vi "Request Data.vi"(6 "Qualifier":string, 8 "error in":errorcluster, 9 "notifier":refnum<notifier>, 10 "Data to Send":string, 11 "Electronic Load in":refnum<class "Electronic Load.lvclass">) -> (0 "error out":errorcluster, 3 "Electronic Load out":refnum<class "Electronic Load.lvclass">)   [LabVIEW 2019, in "Electronic Load.lvlib" / "Electronic Load.lvclass"]
uses:
  Library/Electronic Load.lvclass
  C:/Users/Public/Documents/Development/builds/Instruments/Instruments.lvlibp/Library/Instruments.lvclass
  Library/Electronic Load.lvclass/Electronic Load.ctl
  Accessors/Read Available Channels.vi
  builds/Instruments/Instruments.lvlibp/Accessors/Read Measured.vi
  builds/Instruments/Instruments.lvlibp/Accessors/Read Snapshot.vi
  builds/Instruments/Instruments.lvlibp/Private/Accessors/Read Poll(ms).vi
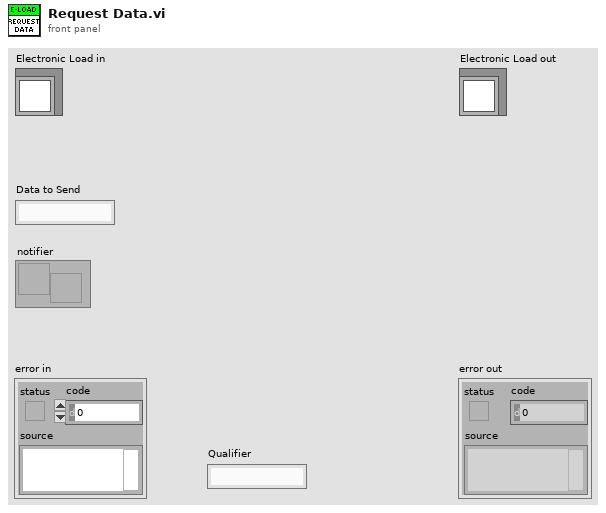
[diagram p1: front panel]
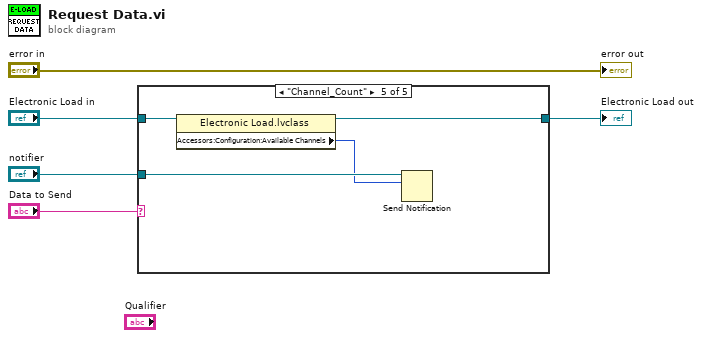
[diagram p0: block diagram]
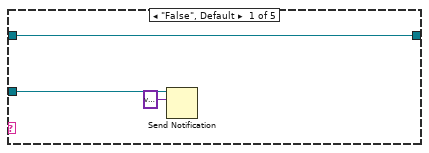
[diagram p2: hidden frame]
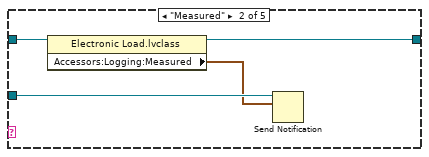
[diagram p3: hidden frame]
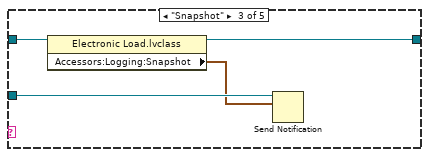
[diagram p4: hidden frame]
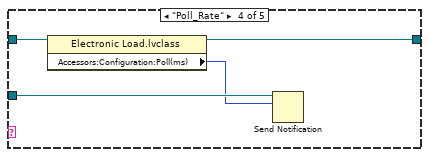
[diagram p5: hidden frame]
diagram:
  n1 = case shown="\"Channel_Count\"" "Data to Send" {
    tunnel: "notifier" -> [w7 w10 w14 w18 w22]
    tunnel: "Electronic Load in" -> [w8 w12 w16 w20 w24]
    tunnel: [w8 w11 w15 w19 w23] -> w1
    frame "False", Default {
      n2 = Send Notification(notification=variant, notifier=w7) -> ()  [unwired: 1 in, 2 out]
    }
    frame "Measured" {
      n3 = property class="Electronic Load.lvclass"(reference=w12) -> (reference out=w11:refnum<class "Electronic Load.lvclass">, "Accessors:Logging:Measured"=w9:waveform(dbl)[])  [unwired: 1 in, 1 out]
      n4 = Send Notification(notification=w9, notifier=w10) -> ()  [unwired: 1 in, 2 out]
    }
    frame "Snapshot" {
      n5 = property class="Electronic Load.lvclass"(reference=w16) -> (reference out=w15:refnum<class "Electronic Load.lvclass">, "Accessors:Logging:Snapshot"=w13:waveform(dbl)[])  [unwired: 1 in, 1 out]
      n6 = Send Notification(notification=w13, notifier=w14) -> ()  [unwired: 1 in, 2 out]
    }
    frame "Poll_Rate" {
      n7 = property class="Electronic Load.lvclass"(reference=w20) -> (reference out=w19:refnum<class "Electronic Load.lvclass">, "Accessors:Configuration:Poll(ms)"=w17:u32)  [unwired: 1 in, 1 out]
      n8 = Send Notification(notification=w17, notifier=w18) -> ()  [unwired: 1 in, 2 out]
    }
    frame "Channel_Count" {
      n9 = property class="Electronic Load.lvclass"(reference=w24) -> (reference out=w23:refnum<class "Electronic Load.lvclass">, "Accessors:Configuration:Available Channels"=w21:i32)  [unwired: 1 in, 1 out]
      n10 = Send Notification(notification=w21, notifier=w22) -> ()  [unwired: 1 in, 2 out]
    }
  }
  "Electronic Load out" <- w1
  "error out" <- "error in"
